vi "gjson_NameFormat.vi"(7 "Encap'd by Array?":bool=TRUE, 8 "error in":errorcluster, 11 "JSON String":string) -> (0 "error out":errorcluster, 3 "JSON_String":string)   [LabVIEW 2015, in "Json2Labv.lvlib"]
doc: "This VI ensures the name is valid. \n(TODO)\n - Conversion to UTF-8\n - Check for escape characters (Maybe not really needed)"
uses:
  Json2Labv.lvlib
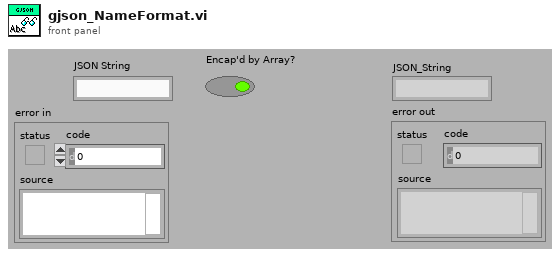
[diagram p1: front panel]
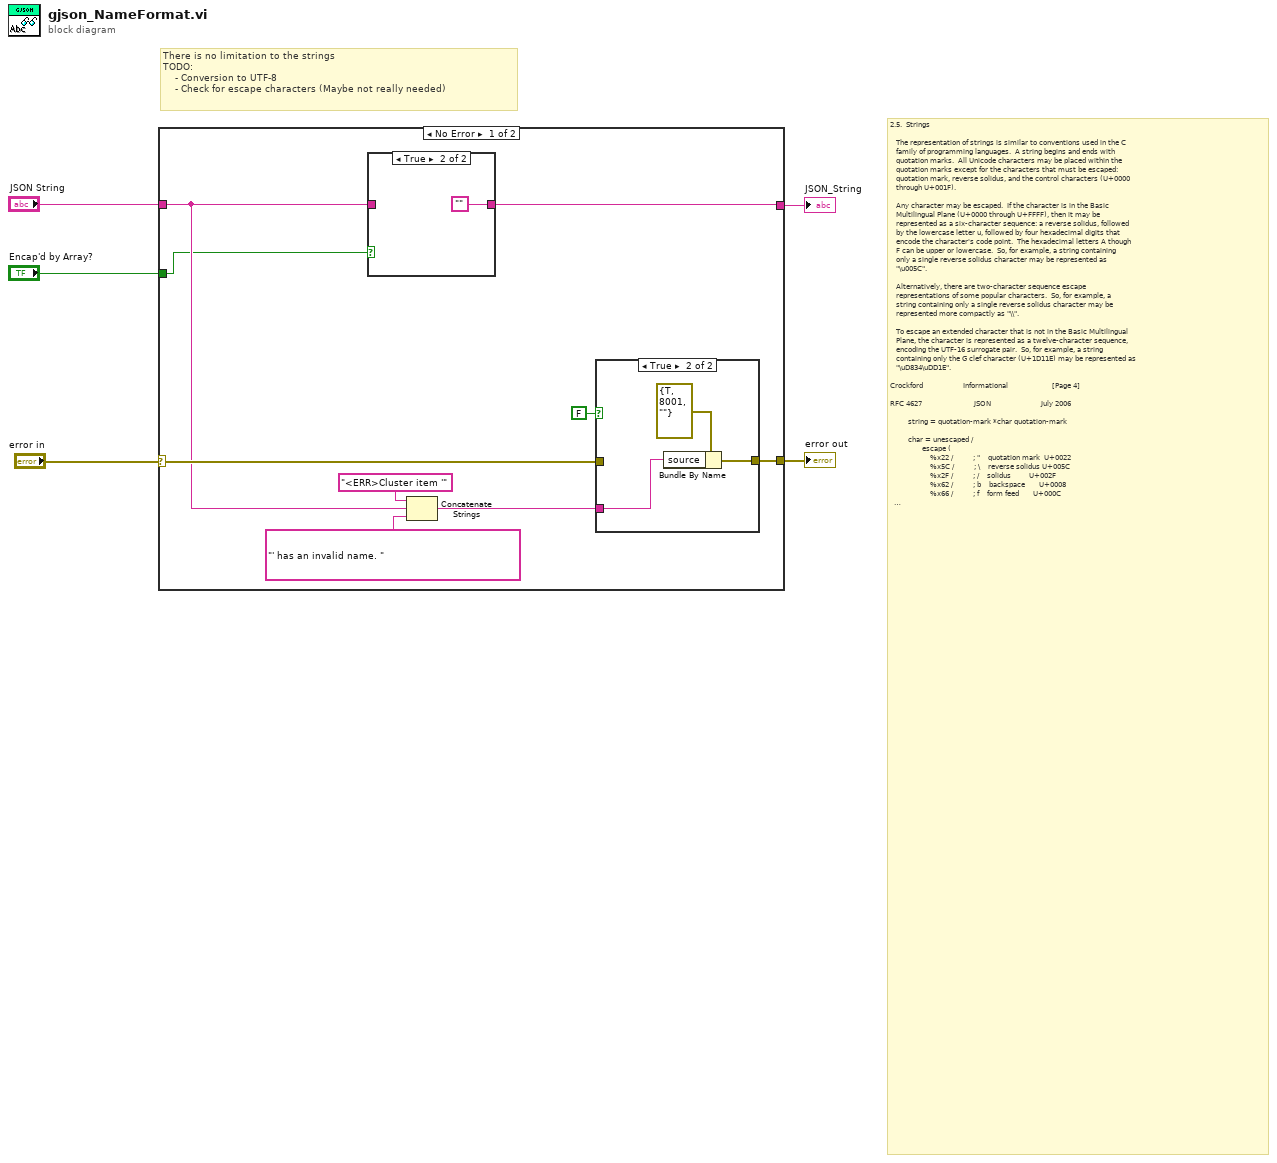
[diagram p0: block diagram]
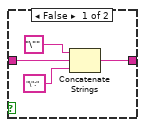
[diagram p2: hidden frame]
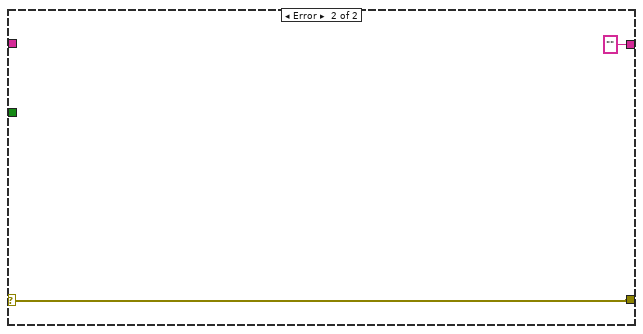
[diagram p4: hidden frame]
diagram:
  # "2.5.  Strings\n\n   The representation of strings is similar to conventions used in the C\n   family of programming languages.  A string begins and ends with\n   quotation marks.  All Unicode characters may be placed within the\n   quotation marks except for the characters that must be escaped:\n   quotation mark, reverse solidus, and the control characters (U+0000\n   through U+001F).\n\n   Any character may be escaped.  If the character is in the Basic\n   Multilingual Plane (U+0000 through U+FFFF), then it may be\n   represented as a six-character sequence: a reverse solidus, followed\n   by the lowercase letter u, followed by four hexadecimal digits that\n   encode the character's code point.  The hexadecimal letters A though\n   F can be upper or lowercase.  So, for example, a string containing\n   only a single reverse solidus character may be represented as\n   \"\\u005C\".\n\n   Alternatively, there are two-character sequence escape\n   representations of some popular characters.  So, for example, a\n   string containing only a single reverse solidus character may be\n   represented more compactly as \"\\\\\".\n\n   To escape an extended character that is not in the Basic Multilingual\n   Plane, the character is represented as a twelve-character sequence,\n   encoding the UTF-16 surrogate pair.  So, for example, a string\n   containing only the G clef character (U+1D11E) may be represented as\n   \"\\uD834\\uDD1E\".\n\nCrockford                    Informational                      [Page 4]\n \nRFC 4627                          JSON                         July 2006\n\n         string = quotation-mark *char quotation-mark\n\n         char = unescaped /\n                escape (\n                    %x22 /          ; \"    quotation mark  U+0022\n                    %x5C /          ; \\    reverse solidus U+005C\n                    %x2F /          ; /    solidus         U+002F\n                    %x62 /          ; b    backspace       U+0008\n                    %x66 /          ; f    form feed       U+000C\n                    %x6E /          ; n    line feed       U+000A\n                    %x72 /          ; r    carriage return U+000D\n                    %x74 /          ; t    tab             U+0009\n                    %x75 4HEXDIG )  ; uXXXX                U+XXXX\n\n         escape = %x5C              ; \\\n\n         quotation-mark = %x22      ; \"\n\n         unescaped = %x20-21 / %x23-5B / %x5D-10FFFF\n\n3.  Encoding\n\n   JSON text SHALL be encoded in Unicode.  The default encoding is\n   UTF-8.\n\n   Since the first two characters of a JSON text will always be ASCII\n   characters [RFC0020], it is possible to determine whether an octet\n   stream is UTF-8, UTF-16 (BE or LE), or UTF-32 (BE or LE) by looking\n   at the pattern of nulls in the first four octets.\n\n           00 00 00 xx  UTF-32BE\n           00 xx 00 xx  UTF-16BE\n           xx 00 00 00  UTF-32LE\n           xx 00 xx 00  UTF-16LE\n           xx xx xx xx  UTF-8"
  # "There is no limitation to the strings \nTODO:\n    - Conversion to UTF-8\n    - Check for escape characters (Maybe not really needed)"
  n1 = case shown="No Error" "error in" {
    selector: "error in" -> [w13 w25]
    tunnel: "JSON String" -> [w8 _]
    tunnel: [w14 w25] -> w4
    tunnel: [w9 "" ("result string")] -> w2
    tunnel: "Encap'd by Array?" -> [w6 _]
    frame No Error {
      n2 = case shown="True" w6 {
        tunnel: [w17 ""] -> w9
        tunnel: w8 -> [w16 _]
        frame False {
          n3 = Concatenate Strings("\"" ("string"), w16, "\":" ("string")) -> (w17:string)
        }
        frame True {
        }
      }
      n4 = Concatenate Strings("<ERR>Cluster item '", w8, "' has an invalid name. ") -> (w11:string)
      n5 = case shown="True" FALSE {
        tunnel: w13 -> [w20 _]
        tunnel: [w20 w22] -> w14
        tunnel: w11 -> [_ w21]
        frame False {
        }
        frame True {
          n6 = Bundle By Name(cluster=errorcluster {"status"=TRUE, "code"=8001, "source"=""} ("error in"), "source"=w21) -> (w22:errorcluster)
        }
      }
    }
    frame Error {
    }
  }
  "error out" <- w4
  "JSON_String" <- w2
